vi "comicvine.to.local_character.vi"(8 "error in (no error)":errorcluster, 11 "cv character":T1) -> (0 "error out":errorcluster, 3 "local character":T5)   [LabVIEW 2024]
uses:
  definitions/local_character.ctl
  definitions/comicvine_character.ctl
  definitions/comicvine_character.results.ctl
  definitions/comicvine_volume.issue.ctl
  definitions/comicvine_volume.publisher.ctl
  <userlib>/_OpenG.lib/string/string.llb/openg_string.lvlib
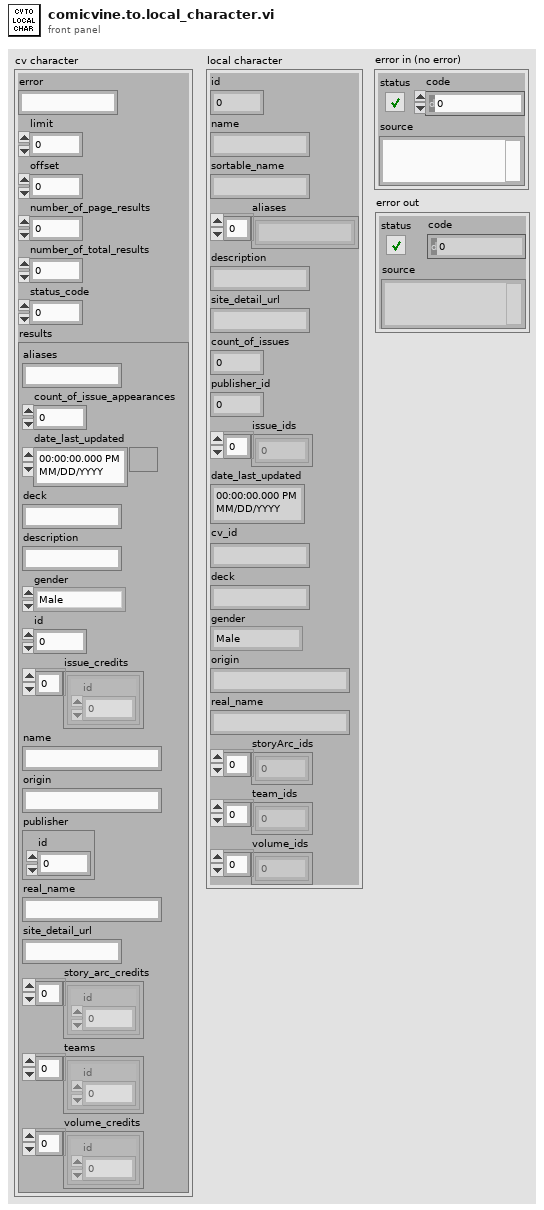
[diagram p1: front panel]
types:
  T1 = typedef "comicvine_character.ctl" = cluster{"error":string, "limit":i32, "offset":i32, "number_of_page_results":i32, "number_of_total_results":i32, "status_code":i32, "results":T2}
  T2 = typedef "comicvine_character.results.ctl" = cluster{"aliases":string, "count_of_issue_appearances":i32, "date_last_updated":timestamp, "deck":string, "description":string, "gender":enum16{"Male", "Female", "Other"}, "id":i32, "issue_credits":T3[], "name":string, "origin":string, "publisher":T4, "real_name":string, "site_detail_url":string, "story_arc_credits":T3[], "teams":T3[], "volume_credits":T3[]}
  T3 = typedef "comicvine_volume.issue.ctl" = cluster{"id":i32}
  T4 = typedef "comicvine_volume.publisher.ctl" = cluster{"id":i32}
  T5 = typedef "local_character.ctl" = cluster{"id":i32, "name":string, "sortable_name":string, "aliases":string[], "description":string, "site_detail_url":string, "count_of_issues":i32, "publisher_id":i32, "issue_ids":i32[], "date_last_updated":timestamp, "cv_id":string, "deck":string, "gender":enum16{"Male", "Female", "Other"}, "origin":string, "real_name":string, "storyArc_ids":i32[], "team_ids":i32[], "volume_ids":i32[]}
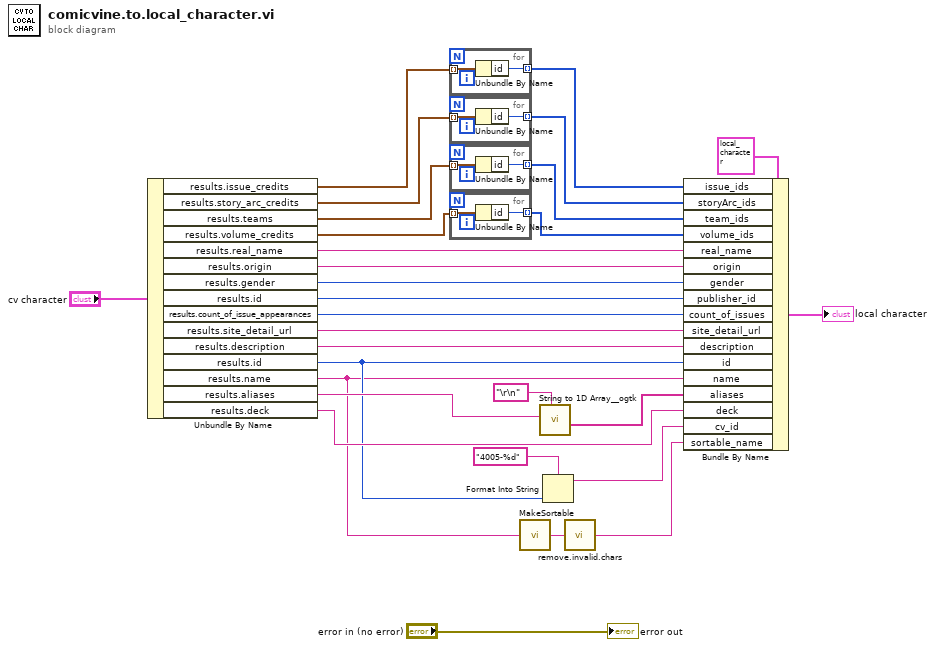
[diagram p0: block diagram]
diagram:
  n1 = Unbundle By Name("cv character") -> ("results.issue_credits"=w6:T3[], "results.story_arc_credits"=w7:T3[], "results.teams"=w8:T3[], "results.volume_credits"=w9:T3[], "results.real_name"=w10:string, "results.origin"=w11:string, "results.gender"=w12:enum16{"Male", "Female", "Other"}, "results.id"=w21:i32, "results.count_of_issue_appearances"=w22:i32, "results.site_detail_url"=w23:string, "results.description"=w24:string, "results.id"=w18:i32, "results.name"=w15:string, "results.aliases"=w27:string, "results.deck"=w20:string)
  n2 = for {
    tunnel: w6 -> [w31] mode=indexing
    tunnel: [w30] -> w2 mode=indexing
    n3 = Unbundle By Name(w31) -> ("id"=w30:i32)
  }
  n4 = for {
    tunnel: w7 -> [w33] mode=indexing
    tunnel: [w32] -> w3 mode=indexing
    n5 = Unbundle By Name(w33) -> ("id"=w32:i32)
  }
  n6 = for {
    tunnel: w8 -> [w35] mode=indexing
    tunnel: [w34] -> w4 mode=indexing
    n7 = Unbundle By Name(w35) -> ("id"=w34:i32)
  }
  n8 = for {
    tunnel: w9 -> [w37] mode=indexing
    tunnel: [w36] -> w5 mode=indexing
    n9 = Unbundle By Name(w37) -> ("id"=w36:i32)
  }
  n10 = call "MakeSortable.vi"("string in"=w15) -> ("string out"=w28:string)
  n11 = call <userlib>:"String to 1D Array__ogtk.vi"("delimiter (Tab)"="\r\n", "string"=w27) -> ("Array of Strings"=w25:string[])  [unwired: 9 in]
  n12 = Format Into String(format string="4005-%d", w18) -> (resulting string=w17:string)  [unwired: 2 in, 1 out]
  n13 = call "remove.invalid.chars.vi"("string in"=w28) -> ("string out"=w14:string)
  n14 = Bundle By Name(cluster=T5 {"id"=0, "name"="", "sortable_name"="", "aliases"=[], "description"="", "site_detail_url"="", "count_of_issues"=0, "publisher_id"=0, "issue_ids"=[], "date_last_updated"=timestamp(0 s since 1904-01-01), "cv_id"="", "deck"="", "gender"=enum."Male", "origin"="", "real_name"="", "storyArc_ids"=[], "team_ids"=[], "volume_ids"=[]} ("character"), "issue_ids"=w2, "storyArc_ids"=w3, "team_ids"=w4, "volume_ids"=w5, "real_name"=w10, "origin"=w11, "gender"=w12, "publisher_id"=w21, "count_of_issues"=w22, "site_detail_url"=w23, "description"=w24, "id"=w18, "name"=w15, "aliases"=w25, "deck"=w20, "cv_id"=w17, "sortable_name"=w14) -> (→"local character":T5)
  "error out" <- "error in (no error)"
